vi "Multicolumn_Listbox_set_value.vi"(8 "error in":errorcluster, 10 "MCListbox value (sel index)":i32, 11 "Test-Plan Table (in)":refnum<vi>) -> (0 "error out":errorcluster, 3 "Test-Plan Table (out)":refnum<vi>)   [LabVIEW 2020]
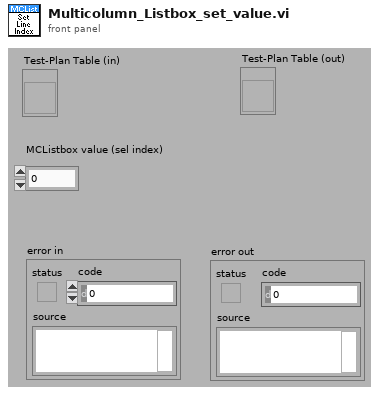
[diagram p1: front panel]
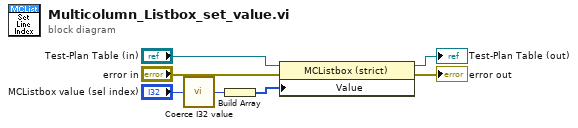
[diagram p0: block diagram]
diagram:
  n1 = call "Coerce I32 value.vi"("I32 value in"="MCListbox value (sel index)") -> ("Coerced value"=w2:i32)  [unwired: 8 in]
  n2 = Build Array(w2) -> (w1:i32[])
  n3 = property on="Property Node" class="MCListbox (strict)"(reference="Test-Plan Table (in)", error in="error in", "Value"=w1) -> (reference out=→"Test-Plan Table (out)":refnum<vi>, error out=→"error out":errorcluster)
